vi "GetConsoleArguments.vi"(6 "error in":errorcluster, 9 "VI Interpreter":refnum<class "VI Interpreter.lvclass">) -> (0 "error out":errorcluster, 3 "VI Interpreter out":refnum<class "VI Interpreter.lvclass">, 4 "outputs":T1[](array[typedef]), 5 "inputs":T1[](array[typedef]))   [LabVIEW 2014, in "Raspberry Pi Compatible Compiler for LabVIEW.lvlib" / "PyConvBD.lvclass"]
uses:
  PyConvBD.lvclass
  VI Interpreter/Classes/VI Interpreter/VI Interpreter.lvclass
  TypeDefs/ConsoleArg_TD.ctl
  VI Interpreter/Classes/Control/Control.lvclass/Control.ctl
  VI Interpreter/Classes/Text/Text.lvclass/Text.ctl
  VI Interpreter/Classes/ControlTerminal/ControlTerminal.lvclass
  VI Interpreter/Classes/Control/Control.lvclass
  VI Interpreter/Classes/Text/Text.lvclass
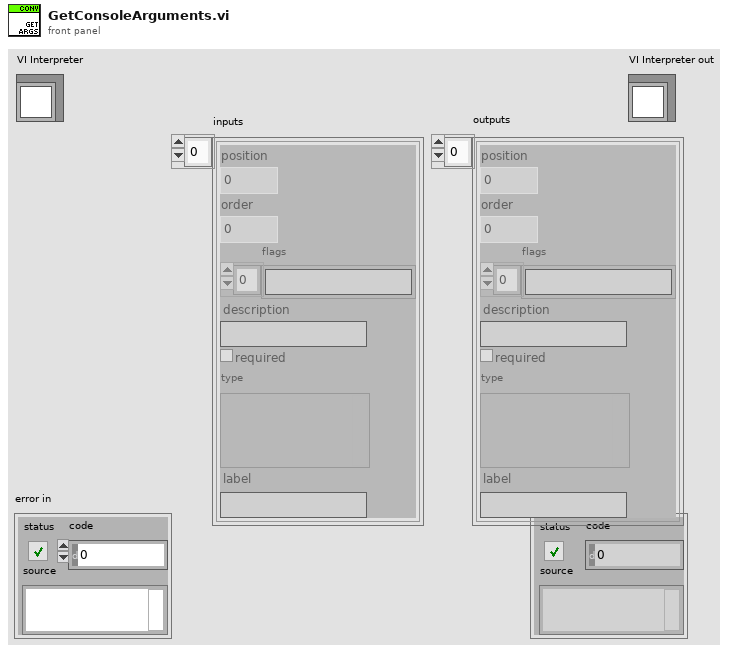
[diagram p1: front panel]
types:
  T1 = typedef "Raspberry Pi Compatible Compiler for LabVIEW.lvlib/PyConvBD.lvclass/ConsoleArg_TD.ctl" = cluster{"position":i32, "order":i32, "flags":string[], "description":string, "required":bool, "type":variant, "label":string}
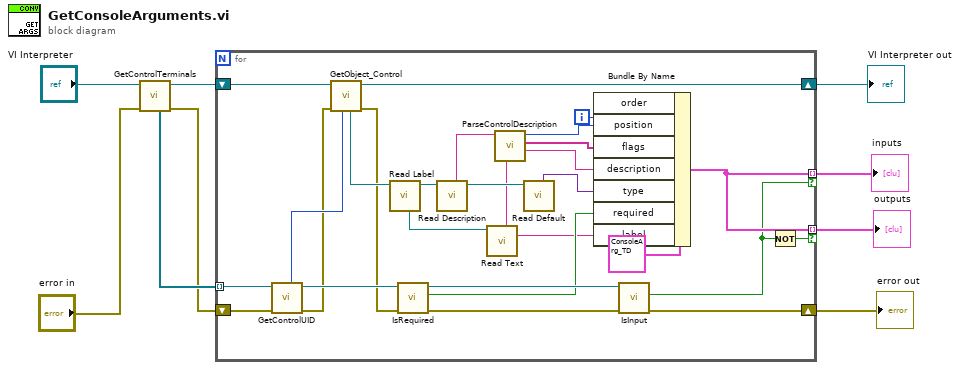
[diagram p0: block diagram]
diagram:
  n1 = call "GetControlTerminals.vi"("error in"="error in", "VI Interpreter in"="VI Interpreter") -> ("error out"=w5:errorcluster, "VI Interpreter out"=w6:refnum<class "VI Interpreter.lvclass">, "controls"=w7:refnum<class "ControlTerminal.lvclass">[])  [unwired: 5 in]
  n2 = for {
    tunnel: w7 -> [w34] mode=indexing
    shift-right: [w15] -> w3
    shift-left: w6 -> [w36]
    shift-right: [w16] -> w4
    shift-left: w5 -> [w33]
    tunnel: [w22] -> w2 mode=indexing if=w21
    tunnel: [w22] -> w1 mode=indexing if=w20
    i -> [w10]
    n3 = call "GetControlUID.vi"("error in"=w33, "Control Terminal in"=w34) -> ("error out"=w19:errorcluster, "Control Terminal out"=w24:refnum<class "ControlTerminal.lvclass">, "control UID"=w35:i32)  [unwired: 5 in]
    n4 = call "GetObject_Control.vi"("UID"=w35, "error in"=w19, "VI Interpreter in"=w36) -> ("error out"=w18:errorcluster, "VI Interpreter out"=w15:refnum<class "VI Interpreter.lvclass">, "control"=w31:refnum<class "Control.lvclass">)  [unwired: 3 in, 1 out]
    n5 = call "Read Label.vi"("Control in"=w31) -> ("Control out"=w30:refnum<class "Control.lvclass">, "Label"=w32:refnum<class "Text.lvclass">)  [unwired: 7 in]
    n6 = call "IsRequired.vi"("error in"=w18, "Control Terminal in"=w24) -> ("error out"=w17:errorcluster, "required"=w14:bool, "Control Terminal out"=w23:refnum<class "ControlTerminal.lvclass">)  [unwired: 7 in]
    n7 = call "Read Description.vi"("Control in"=w30) -> ("Control out"=w13:refnum<class "Control.lvclass">, "Description"=w29:string)  [unwired: 7 in]
    n8 = call "Read Text.vi"("Text in"=w32) -> ("Text"=w11:string)  [unwired: 7 in, 1 out]
    n9 = call "ParseControlDescription.vi"("label"=w11, "Control description"=w29) -> ("description"=w25:string, "flags"=w26:string[], "position"=w27:i32)  [unwired: 5 in]
    n10 = call "Read Default.vi"("Control in"=w13) -> ("Default"=w12:variant)  [unwired: 7 in, 1 out]
    n11 = Bundle By Name(cluster=T1 {"position"=0, "order"=0, "flags"=[], "description"="", "required"=FALSE, "type"=variant, "label"=""}, "order"=w10, "position"=w27, "flags"=w26, "description"=w25, "type"=w12, "required"=w14, "label"=w11) -> (w22:T1)
    n12 = call-dynamic "IsInput.vi"("error in"=w17, "ControlTerminal in"=w23) -> ("error out"=w16:errorcluster, "input"=w21:bool)  [unwired: 5 in, 1 out]
    n13 = Not(x=w21) -> (.not. x?=w20:bool)
  }
  "error out" <- w4
  "VI Interpreter out" <- w3
  "inputs" <- w2
  "outputs" <- w1
